vi "Meas Proc QWTB Update Result View Process.vi"(8 "error in":errorcluster, 11 "session in":variant) -> (0 "error out":errorcluster, 3 "QWTB result session out":variant)   [LabVIEW 2018]
doc: "QWTB result viewer: This VI is async. process that will look into current measurement folder. It scans for results header file, then it reads list of the available results for current QWTB algorithm. It fills the result selector by the list of available results.\nThen it tries to load the result data to the table. It also loads descriptions of the table rows which are stored into the QWTB result session. Alternatively it can generate graph of the selected quantity. The decision table vs graph update is made automatically based on the 'QWTB view setup'."
uses:
  Meas Proc QWTB Plot Legend.ctl
  Meas Proc QWTB Viewer Asyn Session.ctl
  Meas Session.ctl
  adc/ADC Session.ctl
  drivers/niScope/niScope Session.ctl
  drivers/niScope/niScope Virtual Channel Config.ctl
  drivers/niScope/niScope Virtual Channel Mode.ctl
  drivers/niScope/niScope Virtual Channel Input Z.ctl
  drivers/niScope/niScope Virtual Channel Coupling.ctl
  drivers/niScope/niScope Type.ctl
  drivers/niScope/niScope Digitizing Process Options.ctl
  drivers/niScope/niScope Data Packet.ctl
  drivers/niScope/niScope Trigger Setup.ctl
  <instrlib>/niScope/Controls/niScope trigger coupling.ctl
  <instrlib>/niScope/Controls/niScope trigger slope.ctl
  drivers/DMM/3458A Digitizer Session.ctl
  drivers/DMM/3458A Virtual Channel Config.ctl
  drivers/Counter/Counter Session.ctl
  drivers/Counter/Counter Type.ctl
  drivers/AWG/AWG Session.ctl
  drivers/AWG/AWG Type.ctl
  drivers/DMM/3458A Sync Mode.ctl
  drivers/DMM/3458A Idn Mode.ctl
  drivers/DMM/3458A Digitizing Low Levels/Configure/Sampling Mode.ctl
  drivers/DMM/3458A Digitizing Process Options.ctl
  drivers/DMM/3458A Data Packet.ctl
  drivers/DMM/3458A Aux Record Data.ctl
  drivers/DMM/3458A Digitizing Low Levels/Configure/Level Setup.ctl
  drivers/DMM/3458A Digitizing Low Levels/Configure/First Sample Trigger.ctl
  drivers/DMM/3458A Aperture Selection Mode.ctl
  drivers/dsdll/DSDLL Session.ctl
  drivers/dsdll/dsdll source distribution/dsdll_instance.ctl
  drivers/dsdll/dsdll source distribution/dsdll_device_record.ctl
  drivers/dsdll/DSDLL Process Config.ctl
  drivers/dsdll/DSDLL Data Packet.ctl
  adc/ADC Type.ctl
  drivers/simulated_adc/SimAdc Config.ctl
  drivers/simulated_adc/SimAdc Channel Cfg.ctl
  adc/ADC On Close Action.ctl
  drivers/Quatsch_driver/QuADCDriver/QuADC Session.ctl
  drivers/Quatsch_driver/QuADCDriver/QuADC Virtual Channel Config.ctl
  drivers/Quatsch_driver/QuADCDriver/QuADC Virtual Channel Mode.ctl
  drivers/Quatsch_driver/QuADCDriver/QuADC Virtual Channel Input Z.ctl
  drivers/Quatsch_driver/QuADCDriver/QuADC Virtual Channel Coupling.ctl
  drivers/Quatsch_driver/QuADCDriver/QuADC Type.ctl
  drivers/Quatsch_driver/QuADCDriver/QuADC Digitizing Process Options.ctl
  drivers/Quatsch_driver/QuADCDriver/QuADC Data Packet.ctl
  drivers/Quatsch_driver/QuADCDriver/QuADC Trigger Setup.ctl
  Meas Sequence Item.ctl
  Meas Sampling Configuration.ctl
  adc/ADC Trig Config.ctl
  adc/ADC Trig Mode Source.ctl
  adc/ADC Trig Coupling.ctl
  adc/ADC Trig Slope.ctl
  Meas Proc QWTB Algorithm Parameter Data.ctl
  Meas Sequence Configuration.ctl
  Meas Range Mode.ctl
  Meas Sampling Rate Mode.ctl
  octave/golpi/mpc/golpi_session_ref.ctl
  Meas Process Config.ctl
  Meas Process Mode.ctl
  Meas Process Raw Config.ctl
  Meas Process Raw Result Mode.ctl
  Meas Proc QWTB Setup.ctl
  Meas Proc QWTB Uncertainty Mode.ctl
  Meas Proc QWTB Multicore Setup.ctl
  Meas Proc QWTB Multicore Type.ctl
  Corrections/Corr Setup.ctl
  Corrections/Corr Tranducer Item.ctl
  Corrections/Corr Digitizers.ctl
  Assist/Assist Panel Setup.ctl
  Meas Proc QWTB Viewer References.ctl
  Meas Proc QWTB Update Flags.ctl
  Meas Proc QWTB Plot Config.ctl
  Meas Proc QWTB Plot Scale Mode.ctl
  varilib/SGUI Assign Multiple Strings With Tags By Label.vi
  octave/golpi/GOLPI Library.lvlibp/Private/Get Variable - polymorph parts/Get String.vi
  octave/golpi/GOLPI Library.lvlibp/Private/Get Variable - polymorph parts/Get Double.vi
  octave/golpi/GOLPI Library.lvlibp/Private/Get Variable - polymorph parts/Get 1D Array Double.vi
  octave/golpi/mpc/GOLPI Multi Process.lvlib
  octave/golpi/GOLPI Library.lvlibp
  varilib/varilib.lvlib
  drivers/niScope/niScope Virtual Digitizer.lvlib
  drivers/DMM/3458A Virtual Digitizer.lvlib
  drivers/Counter/Counter.lvlib
  drivers/AWG/AWG.lvlib
  drivers/DMM/3458A Digitizing Low Levels/3458A Digitizing Low Levels.lvlib
  drivers/dsdll/DSDLL Virtual Digitizer.lvlib
  drivers/Quatsch_driver/QuADCDriver/QuADC Virtual Digitizer.lvlib
  drivers/dsdll/dsdll source distribution/dsdll.lvlib
panel:
  out "user session (memory)":path
  in  "Show legend":T1
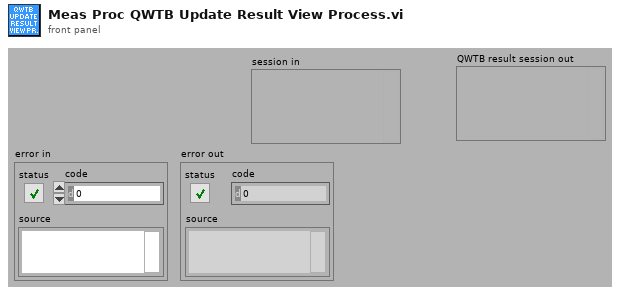
[diagram p1: front panel]
types:
  T1 = typedef "Meas Proc QWTB Plot Legend.ctl" = enum16{"None", "Best", "North", "South", "East", "West", "NorthEast", "NorthWest", "SouthEast", "SouthWest"}
  T2 = typedef "Meas Proc QWTB Viewer Asyn Session.ctl" = cluster{"session":T3, "QWTB result refs":T69, "view setup":T70}
  T3 = typedef "Meas Session.ctl" = cluster{"adc":T4, "sequence":T46[], "sequence setup":T53, "golpi":T56, "processing setup":T57, "corrections":T65, "assist cfg":T68}
  T4 = typedef "ADC Session.ctl" = cluster{"niScope":T5, "3458A":T15, "dsdll":T30, "type":T34, "channel idn str":string[], "aux instr idn str":string[], "modified?":bool, "simadc":T35, "force rst?":bool, "exit mode":T37, "exit dly":dbl, "exit tmr":timestamp, "busy?":bool, "accessed?":bool, "QuADC session":T38}
  T5 = typedef "niScope Virtual Digitizer.lvlib/niScope Session.ctl" = cluster{"channel cfg":T6[], "sessions":refnum<k20>[], "multi cards":bool, "channels":i32, "type":T10, "memory [B/chn]":i32, "ext. clock [Hz]":dbl, "samples count":i64, "use streaming":bool, "proc setup":T11, "sample width [B]":i32, "ranges [V]":dbl[], "trigger setup":T12, "fs [Hz]":dbl, "bitres [bit]":i32}
  T6 = typedef "niScope Virtual Digitizer.lvlib/niScope Virtual Channel Config.ctl" = cluster{"Address":refnum<k15>, "Channel":i32, "Mode":T7, "Input Z":T8, "Coupling":T9, "Range [Vpk]":dbl, "btn clr":bool, "btn up":bool, "btn down":bool}
  T7 = typedef "niScope Virtual Digitizer.lvlib/niScope Virtual Channel Mode.ctl" = enum16{"Single ended", "Unbal. differential", "Differential"}
  T8 = typedef "niScope Virtual Digitizer.lvlib/niScope Virtual Channel Input Z.ctl" = enum16{"1 MOhm", "50 Ohm"}
  T9 = typedef "niScope Virtual Digitizer.lvlib/niScope Virtual Channel Coupling.ctl" = enum16{"AC", "DC", "GND"}
  T10 = typedef "niScope Virtual Digitizer.lvlib/niScope Type.ctl" = enum16{"n/a", "5922"}
  T11 = typedef "niScope Virtual Digitizer.lvlib/niScope Digitizing Process Options.ctl" = cluster{"packet size [smpl]":i64, "current timeout [s]":dbl, "blk2blk timeout [s]":dbl, "event time":timestamp, "temp sampl T [s]":dbl, "data queue":refnum<queue>, "stop notifier":refnum<notifier>, "proc ref":refnum<vi>}
  T12 = typedef "niScope Virtual Digitizer.lvlib/niScope Trigger Setup.ctl" = cluster{"coupling":T13, "level [V]":dbl, "slope":T14, "mode":enum16{"Immediate", "External", "Level"}}
  T13 = typedef "niScope trigger coupling.ctl" = u16
  T14 = typedef "niScope trigger slope.ctl" = i32
  T15 = typedef "3458A Virtual Digitizer.lvlib/3458A Digitizer Session.ctl" = cluster{"channels":T16[], "sync unit":T17, "awg unit":T19, "sync mode":T21, "streaming mode":bool, "idn mode":T22, "sampling mode":T23, "Ts [s]":dbl, "sample memory [B]":i32, "proc setup":T24, "sample size [B]":i32, "sample count":i32, "aux data":T26, "ranges [V]":dbl[], "aperture [s]":dbl, "LEVEL trigger":T27, "trigger mode":T28, "measure temp.?":bool, "disp mesages":string[], "shared bus?":bool, "disable display?":bool, "aper mode":T29, "aper rules":dbl[][]}
  T16 = typedef "3458A Virtual Digitizer.lvlib/3458A Virtual Channel Config.ctl" = cluster{"VISA":refnum<visa-resource-name>, "Range [Vpk]":dbl, "btn clr":bool, "btn up":bool, "btn down":bool}
  T17 = typedef "Counter.lvlib/Counter Session.ctl" = cluster{"VISA":refnum<visa-resource-name>, "type":T18}
  T18 = typedef "Counter.lvlib/Counter Type.ctl" = enum16{"Picotest U6200A", "dummy"}
  T19 = typedef "AWG.lvlib/AWG Session.ctl" = cluster{"type":T20, "VISA":refnum<visa-resource-name>, "enable 10MHz ref":bool}
  T20 = typedef "AWG.lvlib/AWG Type.ctl" = enum16{"Agilent 331xxA to 332xxA", "Agilent 335xxA to 336xxA", "Tektronix AFG3101C", "dummy"}
  T21 = typedef "3458A Virtual Digitizer.lvlib/3458A Sync Mode.ctl" = enum16{"MASTER-SLAVE, MASTER clocked by TIMER", "MASTER-SLAVE, MASTER clocked by AWG", "ALL clocked by AWG", "MASTER-SLAVE, ALL clocked by TIMER", "ALL clocked by AWG with DFLL"}
  T22 = typedef "3458A Virtual Digitizer.lvlib/3458A Idn Mode.ctl" = enum16{"Auto", "Sequential (chn A, chn B, ...)", "From calibration string"}
  T23 = typedef "3458A Virtual Digitizer.lvlib/3458A Digitizing Low Levels.lvlib/Sampling Mode.ctl" = enum16{"DCV", "DSDC", "DSAC"}
  T24 = typedef "3458A Virtual Digitizer.lvlib/3458A Digitizing Process Options.ctl" = cluster{"channel id":i32, "packet size [smpl]":i32, "current timeout [s]":dbl, "blk2blk timeout [s]":dbl, "event time":timestamp, "stop notifier":refnum<notifier>, "data queues":refnum<queue>[], "proc refs":refnum<vi>[], "bus semaphore":T25}
  T25 = typedef "Semaphore RefNum" = refnum<k1>
  T26 = typedef "3458A Virtual Digitizer.lvlib/3458A Aux Record Data.ctl" = cluster{"channel id":i32, "valid?":bool[], "gain [V]":dbl[], "timestamp [s]":dbl[], "Ts [s]":dbl, "abs timestamp":timestamp, "t [deg C]":dbl[]}
  T27 = typedef "3458A Virtual Digitizer.lvlib/3458A Digitizing Low Levels.lvlib/Level Setup.ctl" = cluster{"edge":enum16{"POS", "NEG"}, "level [V]":dbl, "coupling":enum16{"DC", "AC"}}
  T28 = typedef "3458A Virtual Digitizer.lvlib/3458A Digitizing Low Levels.lvlib/First Sample Trigger.ctl" = enum16{"AUTO", "EXT", "SYN", "SGL", "HOLD", "LEVEL"}
  T29 = typedef "3458A Virtual Digitizer.lvlib/3458A Aperture Selection Mode.ctl" = enum16{"Manual", "Maximum", "Table"}
  T30 = typedef "DSDLL Virtual Digitizer.lvlib/DSDLL Session.ctl" = cluster{"dsdll":T31, "channels":i32, "device id":i32, "channel idns":string[], "proc setup":T33, "samples count":i32, "fs [Hz]":dbl}
  T31 = typedef "dsdll.lvlib/dsdll_instance.ctl" = cluster{"dsdll path":path, "dsdll handle":u8[], "output devices":T32[], "capture devices":T32[]}
  T32 = typedef "dsdll.lvlib/dsdll_device_record.ctl" = cluster{"guid":u8[], "name":string}
  T33 = typedef "DSDLL Virtual Digitizer.lvlib/DSDLL Process Config.ctl" = cluster{"packet size [smpl]":i32, "current timeout [s]":dbl, "blk2blk timeout [s]":dbl, "event time":timestamp, "data queue":refnum<queue>, "stop notifier":refnum<notifier>, "proc ref":refnum<vi>}
  T34 = typedef "ADC Type.ctl" = enum16{"niScope", "3458A", "DirectSound DLL", "dummy", "QuADC"}
  T35 = typedef "SimAdc Config.ctl" = cluster{"channels":T36[], "range [V]":dbl, "Ts step [s]":dbl, "time [s]":dbl, "fs [Hz]":dbl, "count":i64, "smpl offset":i64, "set count":i64, "bit res":i32}
  T36 = typedef "SimAdc Channel Cfg.ctl" = cluster{"harmonics":dbl[][], "btn clear":bool, "noise":dbl, "fundamental [Hz]":dbl}
  T37 = typedef "ADC On Close Action.ctl" = enum16{"Immediate reset", "Delayed reset"}
  T38 = typedef "QuADC Virtual Digitizer.lvlib/QuADC Session.ctl" = cluster{"channel cfg":T39[], "sessions":refnum<k5>[], "multi cards":bool, "channels":i32, "type":T43, "memory [B/chn]":i32, "ext. clock [Hz]":dbl, "samples count":i64, "use streaming":bool, "proc setup":T44, "sample width [B]":i32, "ranges [V]":dbl[], "trigger setup":T45, "fs [Hz]":dbl, "bitres [bit]":i32}
  T39 = typedef "QuADC Virtual Digitizer.lvlib/QuADC Virtual Channel Config.ctl" = cluster{"Channel":i32, "Mode":T40, "Input Z":T41, "Coupling":T42, "Range [Vpk]":dbl, "btn clr":bool, "btn up":bool, "btn down":bool, "IP address A":u8, "IP address B":u8, "IP address C":u8, "IP address D":u8, "Port":u16, "Number of JJ":u32, "Clock fr. (Hz)":dbl}
  T40 = typedef "QuADC Virtual Digitizer.lvlib/QuADC Virtual Channel Mode.ctl" = enum16{"Single ended", "Unbal. differential", "Differential"}
  T41 = typedef "QuADC Virtual Digitizer.lvlib/QuADC Virtual Channel Input Z.ctl" = enum16{"1 MOhm", "50 Ohm"}
  T42 = typedef "QuADC Virtual Digitizer.lvlib/QuADC Virtual Channel Coupling.ctl" = enum16{"AC", "DC", "GND"}
  T43 = typedef "QuADC Virtual Digitizer.lvlib/QuADC Type.ctl" = enum16{"n/a", "v1"}
  T44 = typedef "QuADC Virtual Digitizer.lvlib/QuADC Digitizing Process Options.ctl" = cluster{"packet size [smpl]":i64, "current timeout [s]":dbl, "blk2blk timeout [s]":dbl, "event time":timestamp, "temp sampl T [s]":dbl, "data queue":refnum<queue>, "stop notifier":refnum<notifier>, "proc ref":refnum<vi>}
  T45 = typedef "QuADC Virtual Digitizer.lvlib/QuADC Trigger Setup.ctl" = cluster{"coupling":T13, "level [V]":dbl, "slope":T14, "mode":enum16{"Immediate", "External", "Level"}}
  T46 = typedef "Meas Sequence Item.ctl" = cluster{"config":T47, "data file path":path, "header file path":path, "group id":i32, "average id":i32, "group done?":bool, "adc modified?":bool, "source modified?":bool, "progress [%]":dbl, "groups cnt":i32, "average cnt":i32, "data file relative path":string, "meas root path":path, "calculate?":bool}
  T47 = typedef "Meas Sampling Configuration.ctl" = cluster{"fs [Hz]":dbl, "count [smpl]":i64, "aperture [s]":dbl, "trigger":T48, "ranges [Vpk]":dbl[], "QWTB parameters":T52[]}
  T48 = typedef "ADC Trig Config.ctl" = cluster{"source":T49, "level [V]":dbl, "coupling":T50, "slope":T51}
  T49 = typedef "ADC Trig Mode Source.ctl" = enum16{"Immediate", "External", "Level"}
  T50 = typedef "ADC Trig Coupling.ctl" = enum16{"DC", "AC"}
  T51 = typedef "ADC Trig Slope.ctl" = enum16{"POS", "NEG"}
  T52 = typedef "Meas Proc QWTB Algorithm Parameter Data.ctl" = cluster{"name":string, "numerics":dbl[], "strings":string[]}
  T53 = typedef "Meas Sequence Configuration.ctl" = cluster{"group setups":T47[], "average cycles":i32, "range mode":T54, "fs mode":T55, "rng even":dbl, "rng odd":dbl, "folder":path, "name base":string, "meas id":i32, "settle [s]":dbl}
  T54 = typedef "Meas Range Mode.ctl" = enum16{"Keep defaults", "Set All channels", "Set Odd and Even channels"}
  T55 = typedef "Meas Sampling Rate Mode.ctl" = enum16{"Frequency", "Period"}
  T56 = typedef "GOLPI Multi Process.lvlib/golpi_session_ref.ctl" = refnum<vi>
  T57 = typedef "Meas Process Config.ctl" = cluster{"mode":T58, "call after avgs?":bool, "calculate?":bool, "raw mode":T59, "QWTB":T61}
  T58 = typedef "Meas Process Mode.ctl" = enum16{"Raw", "QWTB"}
  T59 = typedef "Meas Process Raw Config.ctl" = cluster{"command":string, "result mode":T60, "res variable":string}
  T60 = typedef "Meas Process Raw Result Mode.ctl" = enum16{"Display console output (only Octave)", "Display string variable", "Display result file %respath%"}
  T61 = typedef "Meas Proc QWTB Setup.ctl" = cluster{"QWTB path":path, "alg filter path":string, "alg ids":string[], "alg parameters":string[], "parsed parameters":T52[], "selected alg id":string, "selected unc mode":T62, "qwtb mcc":i32, "qwtb timeout":i32, "qwtb covg":dbl, "qwtb ofs":i64, "qwtb lim data":i64, "multicore":T63, "unc once?":bool}
  T62 = typedef "Meas Proc QWTB Uncertainty Mode.ctl" = enum16{"None", "GUF", "Monte Carlo"}
  T63 = typedef "Meas Proc QWTB Multicore Setup.ctl" = cluster{"jobs folder":path, "cores":i32, "max jobs":i32, "mode":T64}
  T64 = typedef "Meas Proc QWTB Multicore Type.ctl" = enum16{"Singlecore", "Multicore", "Multistation"}
  T65 = typedef "Corr Setup.ctl" = cluster{"transducers":cluster{"channels":T66[], "last path":path}, "digitizer":T67}
  T66 = typedef "Corr Tranducer Item.ctl" = cluster{"Path":path, "Ratio:":string, "Name:":string, "btn rem":bool, "btn up":bool, "btn down":bool, "s.n.:":string, "btn open":bool, "ratio o/i":dbl, "chn hi":u16, "chn lo":u16, "Phase index":i32}
  T67 = typedef "Corr Digitizers.ctl" = cluster{"last path":path, "channel paths":path[], "channel idns":string[], "correction name":string, "channel names":string[], "folders to copy":path[], "channel valid":bool[], "correction path":path, "correction rel path":string, "rel folders to copy":string[]}
  T68 = typedef "Assist Panel Setup.ctl" = cluster{"P":i32, "Q":i32, "rel shift":dbl, "ref freq":dbl, "min fs":dbl, "max fs tol":dbl, "min int":dbl, "max int":dbl, "max err":dbl, "max timeout":dbl}
  T69 = typedef "Meas Proc QWTB Viewer References.ctl" = cluster{"tc result":refnum<vi>, "qwtb results tbl":refnum<vi>, "qwtb maxdim":refnum<vi>, "qwtb unc":refnum<vi>, "qwtb order":refnum<vi>, "qwtb maxarr":refnum<vi>, "qwtb res sel":refnum<vi>, "qwtb res info":refnum<vi>, "descriptions":string[], "var names":string[], "channel indexes":i32[], "qwtb ref chn":refnum<vi>, "qwtb ph unit":refnum<vi>, "qwtb alg sel":refnum<vi>, "qwtb meas sel":refnum<vi>, "qwtb ssn info":refnum<vi>, "last session":path, "qwtb qu list":refnum<vi>}
  T70 = typedef "Meas Proc QWTB Update Flags.ctl" = cluster{"new result":bool, "show graph":bool, "plot setup":T71, "new session":bool}
  T71 = typedef "Meas Proc QWTB Plot Config.ctl" = cluster{"X-axis style":T72, "Y-axis style":T72, "Show legend":T1, "Grid on":bool, "Box on":bool, "show all chn":bool}
  T72 = typedef "Meas Proc QWTB Plot Scale Mode.ctl" = enum16{"Linear", "Log"}
  T73 = typedef "GOLPI Library.lvlibp/GOLPI reference Type Def.ctl" = cluster{"pipe handle":T74, "fast read timeout [ms]":u32, "fast read settle time [ms]":u32, "fast read to multiple [ms]":u32, "max elements per input line":u32, "slow read timeout [ms]":u32, "stdin double format specifier":string, "max elements per stdout output column":u32, "console mode bitstream":bool, "bitstream first read timeout [ms]":u32, "bitstream read timeout [ms]":u32, "struct transfer possible":bool, "matlab mode":bool}
  T74 = typedef "GOLPI Library.lvlibp/LV Process library.lvlib/Pipe Handle.ctl" = cluster{"lv_proc.dll file path":path, "process instance handle":u32[], "debug mode":bool, "debug data":cluster{"time":timestamp, "stdin":bool, "data":string}[]}
  T75 = typedef "Meas Proc QWTB View Max Dim.ctl" = enum16{"Scalar", "Vector", "Matrix"}
  T76 = typedef "Meas Proc QWTB View Group Mode.ctl" = enum16{"Group quantities", "Group phases"}
  T77 = typedef "Meas Proc QWTB View Uncertainty Mode.ctl" = enum16{"None", "val ± unc", "[val; unc]"}
  T78 = typedef "Meas Proc QWTB View Phase Mode.ctl" = enum16{"± pi [rad]", "0 - 2*pi [rad]", "±180 [deg]", "0 - 360 [deg]"}
  T79 = typedef "LVRowAndColumnTypeDef.ctl" = cluster{"Row":i32, "Column":i32}
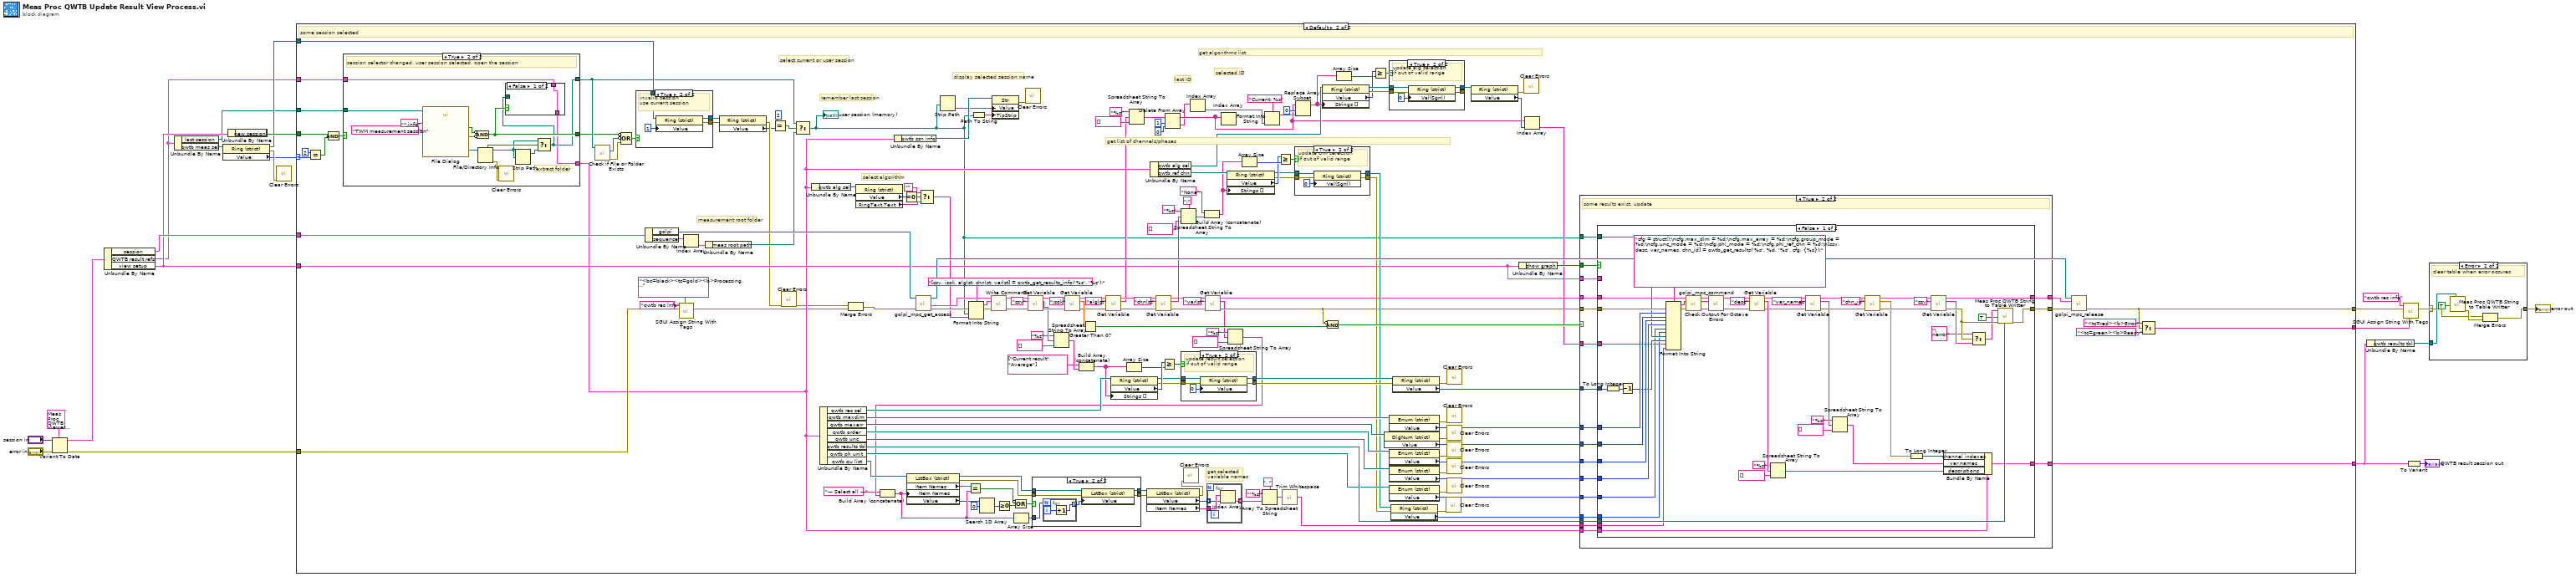
[diagram p0: block diagram]
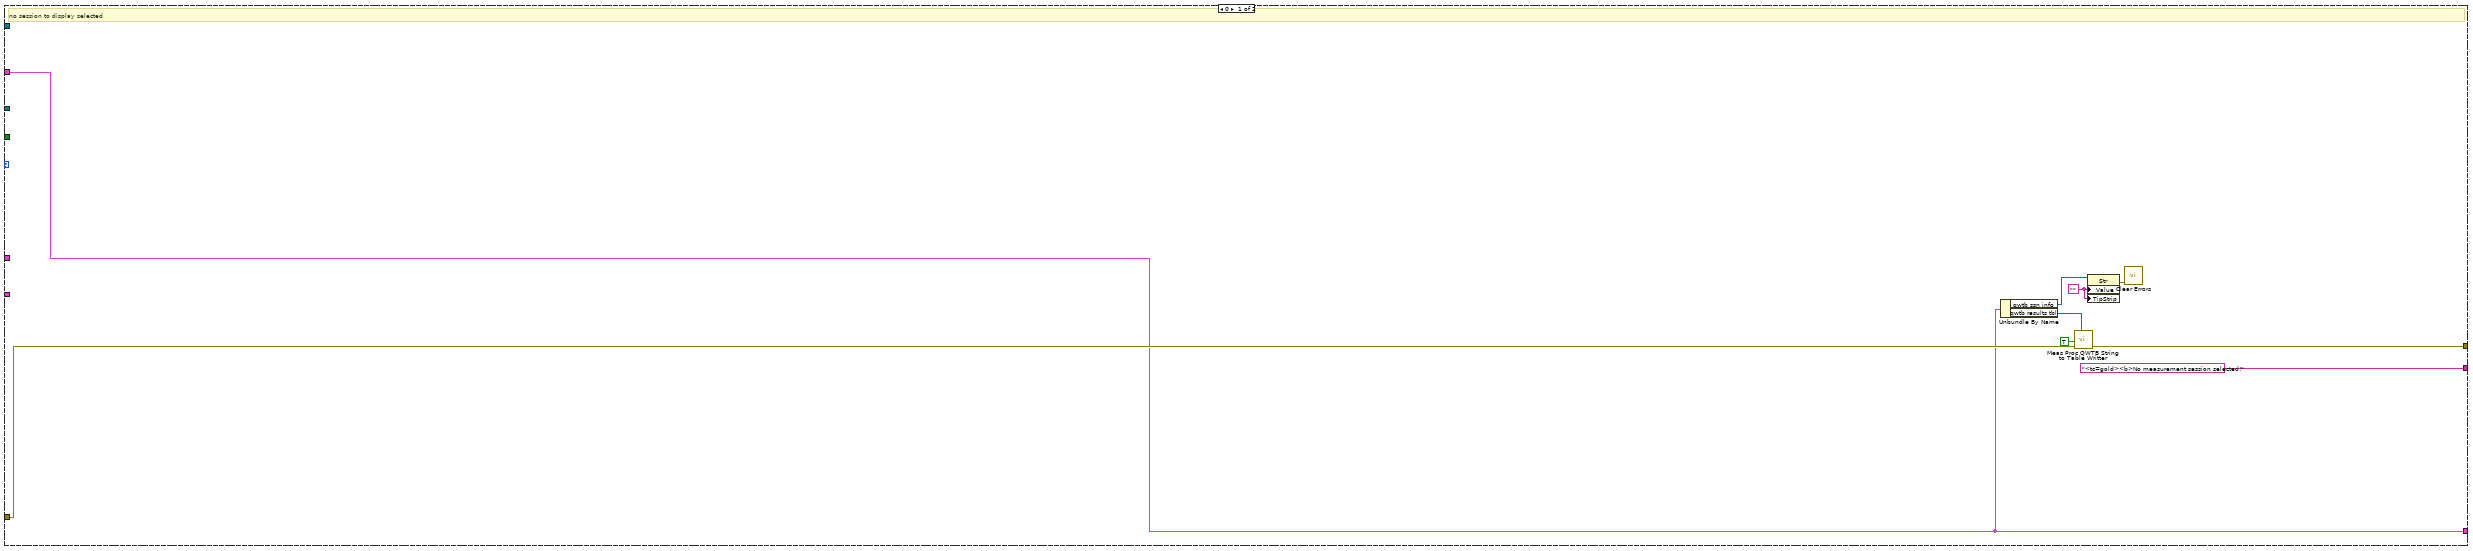
[diagram p3: hidden frame]
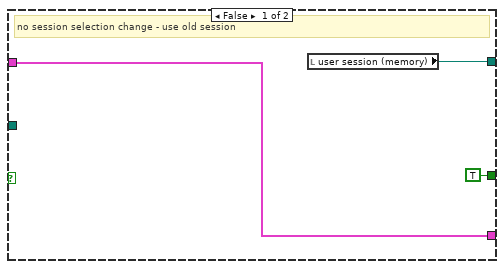
[diagram p6: hidden frame]
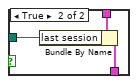
[diagram p7: hidden frame]
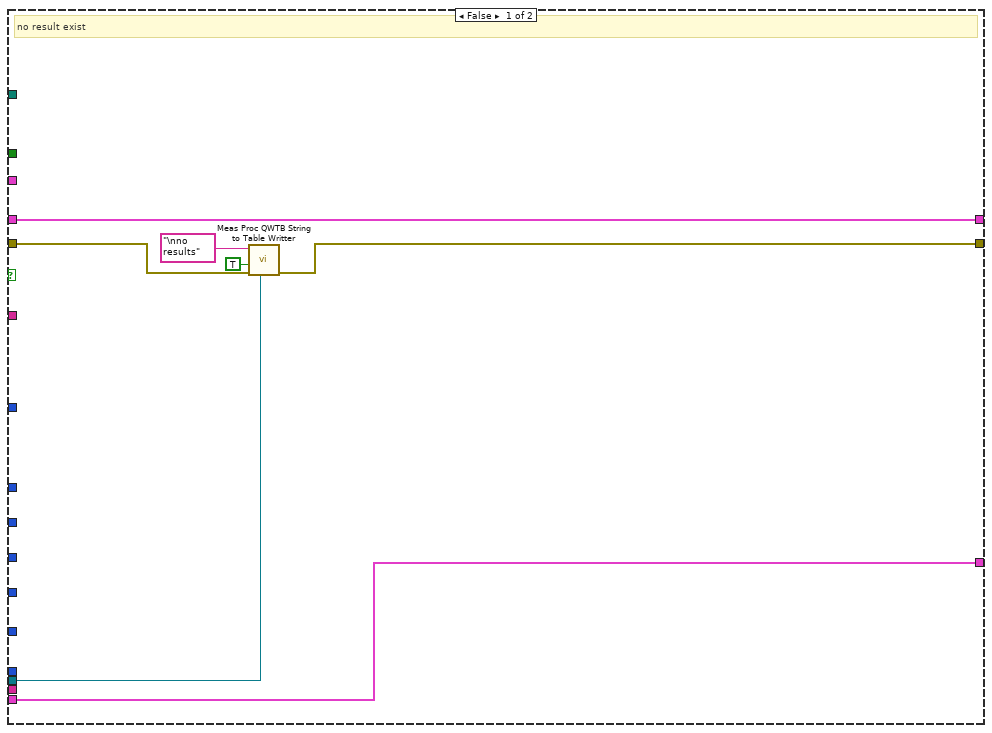
[diagram p10: hidden frame]
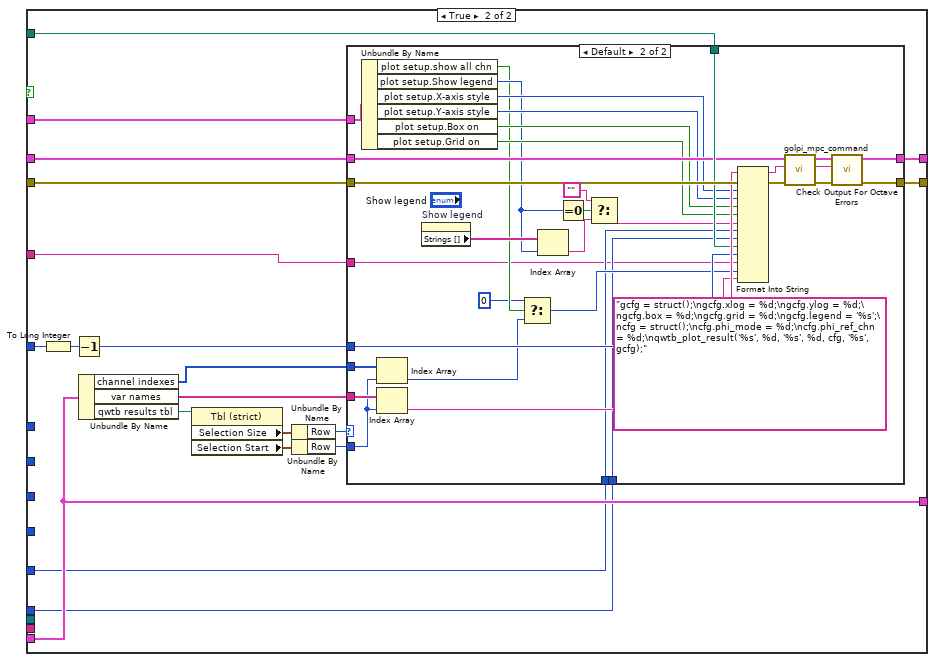
[diagram p11: hidden frame]
diagram:
  n1 = Variant To Data(error in="error in", type=T2 {"session"={"adc"={"niScope"={"channel cfg"=[], "sessions"=[], "multi cards"=FALSE, "channels"=0, "type"=enum."n/a", "memory [B/chn]"=0, "ext. clock [Hz]"=0.0, "samples count"=0, "use streaming"=FALSE, "proc setup"={"packet size [smpl]"=0, "current timeout [s]"=0.0, "blk2blk timeout [s]"=0.0, "event time"=timestamp(0 s since 1904-01-01), "temp sampl T [s]"=0.0, "data queue"=refnum, "stop notifier"=refnum, "proc ref"=refnum}, "sample width [B]"=0, "ranges [V]"=[], "trigger setup"={"coupling"=1, "level [V]"=0.0, "slope"=0, "mode"=enum."Immediate"}, "fs [Hz]"=0.0, "bitres [bit]"=0}, "3458A"={"channels"=[], "sync unit"={"VISA"="", "type"=enum."Picotest U6200A"}, "awg unit"={"type"=enum."Agilent 331xxA to 332xxA", "VISA"="", "enable 10MHz ref"=FALSE}, "sync mode"=enum."MASTER-SLAVE, MASTER clocked by TIMER", "streaming mode"=FALSE, "idn mode"=enum."Auto", "sampling mode"=enum."DCV", "Ts [s]"=0.0, "sample memory [B]"=0, "proc setup"={"channel id"=0, "packet size [smpl]"=0, "current timeout [s]"=0.0, "blk2blk timeout [s]"=0.0, "event time"=timestamp(0 s since 1904-01-01), "stop notifier"=refnum, "data queues"=[], "proc refs"=[], "bus semaphore"=refnum}, "sample size [B]"=0, "sample count"=0, "aux data"={"channel id"=0, "valid?"=[], "gain [V]"=[], "timestamp [s]"=[], "Ts [s]"=0.0, "abs timestamp"=timestamp(0 s since 1904-01-01), "t [deg C]"=[]}, "ranges [V]"=[], "aperture [s]"=0.0, "LEVEL trigger"={"edge"=enum."POS", "level [V]"=0.0, "coupling"=enum."DC"}, "trigger mode"=enum."AUTO", "measure temp.?"=FALSE, "disp mesages"=[], "shared bus?"=FALSE, "disable display?"=FALSE, "aper mode"=enum."Manual", "aper rules"=[]}, "dsdll"={"dsdll"={"dsdll path"=path "", "dsdll handle"=[], "output devices"=[], "capture devices"=[]}, "channels"=0, "device id"=0, "channel idns"=[], "proc setup"={"packet size [smpl]"=0, "current timeout [s]"=0.0, "blk2blk timeout [s]"=0.0, "event time"=timestamp(0 s since 1904-01-01), "data queue"=refnum, "stop notifier"=refnum, "proc ref"=refnum}, "samples count"=0, "fs [Hz]"=0.0}, "type"=enum."niScope", "channel idn str"=[], "aux instr idn str"=[], "modified?"=FALSE, "simadc"={"channels"=[], "range [V]"=0.0, "Ts step [s]"=0.0, "time [s]"=0.0, "fs [Hz]"=0.0, "count"=0, "smpl offset"=0, "set count"=0, "bit res"=0}, "force rst?"=FALSE, "exit mode"=enum."Immediate reset", "exit dly"=0.0, "exit tmr"=timestamp(0 s since 1904-01-01), "busy?"=FALSE, "accessed?"=FALSE, "QuADC session"={"channel cfg"=[], "sessions"=[], "multi cards"=FALSE, "channels"=0, "type"=enum."n/a", "memory [B/chn]"=0, "ext. clock [Hz]"=0.0, "samples count"=0, "use streaming"=FALSE, "proc setup"={"packet size [smpl]"=0, "current timeout [s]"=0.0, "blk2blk timeout [s]"=0.0, "event time"=timestamp(0 s since 1904-01-01), "temp sampl T [s]"=0.0, "data queue"=refnum, "stop notifier"=refnum, "proc ref"=refnum}, "sample width [B]"=0, "ranges [V]"=[], "trigger setup"={"coupling"=0, "level [V]"=0.0, "slope"=0, "mode"=enum."Immediate"}, "fs [Hz]"=0.0, "bitres [bit]"=0}}, "sequence"=[], "sequence setup"={"group setups"=[], "average cycles"=0, "range mode"=enum."Keep defaults", "fs mode"=enum."Frequency", "rng even"=0.0, "rng odd"=0.0, "folder"=path "", "name base"="", "meas id"=0, "settle [s]"=0.0}, "golpi"=refnum, "processing setup"={"mode"=enum."Raw", "call after avgs?"=FALSE, "calculate?"=FALSE, "raw mode"={"command"="", "result mode"=enum."Display console output (only Octave)", "res variable"=""}, "QWTB"={"QWTB path"=path "", "alg filter path"="", "alg ids"=[], "alg parameters"=[], "parsed parameters"=[], "selected alg id"="", "selected unc mode"=enum."None", "qwtb mcc"=0, "qwtb timeout"=0, "qwtb covg"=0.0, "qwtb ofs"=0, "qwtb lim data"=0, "multicore"={"jobs folder"=path "", "cores"=0, "max jobs"=0, "mode"=enum."Singlecore"}, "unc once?"=FALSE}}, "corrections"={"transducers"={"channels"=[], "last path"=path ""}, "digitizer"={"last path"=path "", "channel paths"=[], "channel idns"=[], "correction name"="", "channel names"=[], "folders to copy"=[], "channel valid"=[], "correction path"=path "", "correction rel path"="", "rel folders to copy"=[]}}, "assist cfg"={"P"=0, "Q"=0, "rel shift"=0.0, "ref freq"=0.0, "min fs"=0.0, "max fs tol"=0.0, "min int"=0.0, "max int"=0.0, "max err"=0.0, "max timeout"=0.0}}, "QWTB result refs"={"tc result"=refnum, "qwtb results tbl"=refnum, "qwtb maxdim"=refnum, "qwtb unc"=refnum, "qwtb order"=refnum, "qwtb maxarr"=refnum, "qwtb res sel"=refnum, "qwtb res info"=refnum, "descriptions"=[], "var names"=[], "channel indexes"=[], "qwtb ref chn"=refnum, "qwtb ph unit"=refnum, "qwtb alg sel"=refnum, "qwtb meas sel"=refnum, "qwtb ssn info"=refnum, "last session"=path "", "qwtb qu list"=refnum}, "view setup"={"new result"=FALSE, "show graph"=FALSE, "plot setup"={"X-axis style"=enum."Linear", "Y-axis style"=enum."Linear", "Show legend"=enum."None", "Grid on"=FALSE, "Box on"=FALSE, "show all chn"=FALSE}, "new session"=FALSE}} ("Cluster"), Variant="session in") -> (data=w18:T2, error out=w16:errorcluster)
  n2 = Unbundle By Name(w18) -> ("session"=w17:T3, "QWTB result refs"=w9:T69, "view setup"=w15:T70)
  n3 = Unbundle By Name(w9) -> ("last session"=w10:path, "qwtb meas sel"=w14:refnum<vi>)
  n4 = property class="Ring (strict)"(reference=w14) -> (reference out=w12:refnum<vi>, error out=w11:errorcluster, "Value"=w8:u16)  [unwired: 1 in]
  n5 = Unbundle By Name(w15) -> ("new session"=w13:bool)
  n6 = call <vilib>:"Clear Errors.vi"("error in (no error)"=w11) -> ()  [unwired: 5 in, 2 out]
  n7 = case shown="Default" w8 {
    selector: w8 -> [_ w73]
    tunnel: [w29 w72] -> w6
    tunnel: [w28 w64] -> w2
    tunnel: w17 -> [_ w150]
    tunnel: w16 -> [w30 w149]
    tunnel: w15 -> [_ w102]
    tunnel: w13 -> [_ w101]
    tunnel: w12 -> [_ w97]
    tunnel: w10 -> [_ w86]
    tunnel: w9 -> [w28 w85]
    tunnel: ["<tc=gold><b>No measurement session selected!" ("string (empty)") w71] -> w5
    frame 0 {
      w24 = "" ("Value")
      # "no session to display selected"
      n8 = Unbundle By Name(w28) -> ("qwtb ssn info"=w25:refnum<vi>, "qwtb results tbl"=w27:refnum<vi>)
      n9 = call "Meas Proc QWTB String to Table Writter.vi"("param table ref"=w27, "error in"=w30, "force data update? (False)"=TRUE) -> ("error out"=w29:errorcluster)  [unwired: 7 in, 1 out]
      n10 = property class="Str"(reference=w25, "Value"=w24, "TipStrip"=w24) -> (error out=w23:errorcluster)  [unwired: 1 in, 1 out]
      n11 = call <vilib>:"Clear Errors.vi"("error in (no error)"=w23) -> ()  [unwired: 5 in, 2 out]
    }
    frame Default {
      # "get selected\nvariable names"
      # "last ID"
      # "selected ID"
      # "display selected session name"
      # "remember last session"
      # "select current or user session"
      # "select algorithm"
      # "get list of channels/phases"
      # "get algorithms list"
      # "measurement root folder"
      # "some session selected"
      n12 = Equal?(x=u16 2, y=w73) -> (x = y?=w77:bool)
      n13 = Compound Arithmetic op=AND(w101, w77) -> (w100:bool)
      n14 = case shown="True" w100 {
        tunnel: [w228 w230] -> w96
        tunnel: [TRUE w231] -> w95
        tunnel: w86 -> [_ w232]
        tunnel: w85 -> [w226 w233]
        tunnel: [w226 w229] -> w84
        frame False {
          # "no session selection change - use old session"
          n15 = local read "user session (memory)"() -> (w228:path)
        }
        frame True {
          # "extract folder"
          # "session selector changed, user session selected, open the session"
          n16 = call "File Dialog"("start path"=w232, "pattern (all files)"="*.info", "pattern label"="TWM measurement session") -> ("selected path"=w238:path, "cancelled"=w240:bool, "error out"=w239:errorcluster)  [unwired: 9 in, 1 out]
          n17 = Compound Arithmetic op=AND(invert w240, invert w239) -> (w231:bool)
          n18 = File/Directory Info(path=w238) -> (path out=w236:path, directory=w237:bool, error out=w234:errorcluster)  [unwired: 1 in, 4 out]
          n19 = call <vilib>:"Clear Errors.vi"("error in (no error)"=w234) -> ()  [unwired: 5 in, 2 out]
          n20 = Strip Path(path=w236) -> (stripped path=w235:path)  [unwired: 1 out]
          n21 = Select(t=w236, s=w237, f=w235) -> (s? t:f=w230:path)
          n22 = case shown="False" w231 {
            tunnel: w233 -> [w243 w246]
            tunnel: w230 -> [_ w245]
            tunnel: [w243 w244] -> w229
            frame False {
            }
            frame True {
              n23 = Bundle By Name(cluster=w246, "last session"=w245) -> (w244:T69)
            }
          }
        }
      }
      n24 = call <vilib>:"Check if File or Folder Exists.vi"("path"=w96) -> ("error out"=w93:errorcluster, "file or folder exists?"=w94:bool)  [unwired: 8 in, 1 out]
      n25 = Compound Arithmetic op=OR(invert w95, invert w94, w93) -> (w92:bool)
      n26 = case shown="True" w92 {
        tunnel: w97 -> [w221 w225]
        tunnel: [w221 w223] -> w98
        tunnel: [_ w222] -> w91
        frame False {
        }
        frame True {
          # "invalid session\nuse current session"
          n27 = property class="Ring (strict)"(reference=w225, "Value"=u16 1) -> (reference out=w223:refnum<vi>, error out=w222:errorcluster)  [unwired: 1 in]
        }
      }
      n28 = Unbundle By Name(w150) -> ("golpi"=w205:T56, "sequence"=w207:T46[])
      n29 = call-poly "SGUI Assign String With Tags.vi"("error in"=w149, "label(s) (empty)"="qwtb res info", "string (empty)"="<bc=black><tc=gold><b>Processing...") -> ("error out"=w83:errorcluster)  [unwired: 7 in, 1 out]
      n30 = Index Array(array=w207) -> (element=w206:T46)  [unwired: 1 in]
      n31 = Unbundle By Name(w206) -> ("meas root path"=w99:path)
      n32 = property class="Ring (strict)"(reference=w98, error in=w91) -> (error out=w90:errorcluster, "Value"=w76:u16)  [unwired: 1 out]
      n33 = Equal?(x=u16 2, y=w76) -> (x = y?=w75:bool)
      n34 = call <vilib>:"Clear Errors.vi"("error in (no error)"=w90) -> ("error out"=w81:errorcluster)  [unwired: 5 in, 1 out]
      n35 = Select(t=w96, s=w75, f=w99) -> (s? t:f=w80:path)
      "user session (memory)" <- w80
      n36 = Unbundle By Name(w84) -> ("qwtb alg sel"=w108:refnum<vi>)
      n37 = Unbundle By Name(w84) -> ("qwtb res sel"=w188:refnum<vi>, "qwtb maxdim"=w174:refnum<vi>, "qwtb maxarr"=w173:refnum<vi>, "qwtb order"=w172:refnum<vi>, "qwtb unc"=w171:refnum<vi>, "qwtb results tbl"=w162:refnum<vi>, "qwtb ph unit"=w152:refnum<vi>, "qwtb qu list"=w48:refnum<vi>)
      n38 = Merge Errors(w81, w83) -> (w82:errorcluster)
      n39 = property class="Ring (strict)"(reference=w108) -> ("Value"=w107:u16, "RingText.Text"=w105:string)  [unwired: 1 in, 2 out]
      n40 = Unbundle By Name(w84) -> ("qwtb ssn info"=w89:refnum<vi>)
      n41 = Equal To 0?(x=w107) -> (x = 0?=w106:bool)
      n42 = call "golpi_mpc_get_access.vi"("error in"=w82, "golpi session ref"=w205) -> ("error out"=w203:errorcluster, "GOLPI ref out"=w204:T73, "golpi session ref out (copy)"=w159:T56)  [unwired: 4 in, 3 out]
      n43 = Select(t="", s=w106, f=w105) -> (s? t:f=w103:string)
      n44 = Strip Path(path=w80) -> (name=w88:string)  [unwired: 1 out]
      n45 = Format Into String(format string="[csv, isok, alglst, chnlst, varlst] = qwtb_get_results_info('%s', '%s');", error in=w203, w80, w103) -> (resulting string=w201:string, error out=w202:errorcluster)  [unwired: 1 in]
      n46 = Path To String(path=w80) -> (string=w79:string)
      n47 = call "Write Command.vi"("error in"=w202, "command"=w201, "GOLPI ref. in"=w204) -> ("error out"=w199:errorcluster, "GOLPI ref. out"=w198:T73)  [unwired: 7 in]
      n48 = property class="Str"(reference=w89, "Value"=w88, "TipStrip"=w79) -> (error out=w87:errorcluster)  [unwired: 1 in, 1 out]
      n49 = call <vilib>:"Clear Errors.vi"("error in (no error)"=w87) -> ()  [unwired: 5 in, 2 out]
      n50 = call-poly "Get Variable.vi"("error in"=w199, "variable name"="csv", "GOLPI ref. in"=w198) -> ("error out"=w196:errorcluster, "value"=w192:string, "GOLPI ref. out"=w194:T73)  [unwired: 6 in]
      n51 = Spreadsheet String To Array(format string="%s", spreadsheet string=w192, array type (2D Dbl)=string[] []) -> (array=w190:string[])  [unwired: 1 in]
      n52 = call-poly "Get Variable.vi"("error in"=w196, "variable name"="isok", "GOLPI ref. in"=w194) -> ("error out"=w130:errorcluster, "value"=w180:dbl, "GOLPI ref. out"=w127:T73)  [unwired: 6 in]
      n53 = Build Array (concatenate)(string[] ["Current result", "Average"], w190) -> (w187:string[])
      n54 = Greater Than 0?(x=w180) -> (x > 0?=w179:bool)
      n55 = call-poly "Get Variable.vi"("error in"=w130, "variable name"="alglst", "GOLPI ref. in"=w127) -> ("error out"=w129:errorcluster, "value"=w123:string, "GOLPI ref. out"=w128:T73)  [unwired: 6 in]
      n56 = property class="Ring (strict)"(reference=w188, "Strings []"=w187) -> (reference out=w183:refnum<vi>, error out=w182:errorcluster, "Value"=w186:u16)  [unwired: 1 in]
      n57 = Array Size(array=w187) -> (size(s)=w185:i32)
      n58 = Spreadsheet String To Array(format string="%s", spreadsheet string=w123, array type (2D Dbl)=string[] []) -> (array=w70:string[])  [unwired: 1 in]
      n59 = Unbundle By Name(w84) -> ("qwtb alg sel"=w113:refnum<vi>, "qwtb ref chn"=w141:refnum<vi>)
      n60 = call-poly "Get Variable.vi"("error in"=w129, "variable name"="chnlst", "GOLPI ref. in"=w128) -> ("error out"=w56:errorcluster, "value"=w145:string, "GOLPI ref. out"=w54:T73)  [unwired: 6 in]
      n61 = Greater Or Equal?(x=w186, y=w185) -> (x >= y?=w184:bool)
      n62 = Delete From Array(array=w70, length=1, index=0) -> (deleted portion=w67:string[], array with subset deleted=w69:string[])
      n63 = Spreadsheet String To Array(delimiter (Tab)=";", format string="%s", spreadsheet string=w145, array type (2D Dbl)=string[] []) -> (array=w140:string[])
      n64 = case shown="True" w184 {
        tunnel: w183 -> [w393 w399]
        tunnel: w182 -> [w394 w398]
        tunnel: [w394 w396] -> w178
        tunnel: [w393 w395] -> w177
        frame False {
        }
        frame True {
          # "update result selection\nif out of valid range"
          n65 = property class="Ring (strict)"(reference=w399, error in=w398, "Value"=u16 0) -> (reference out=w395:refnum<vi>, error out=w396:errorcluster)
        }
      }
      n66 = Index Array(array=w67) -> (element=w66:string)  [unwired: 1 in]
      n67 = Build Array (concatenate)("None" ("delimiter (Tab)"), w140) -> (w138:string[])
      n68 = call-poly "Get Variable.vi"("error in"=w56, "variable name"="varlst", "GOLPI ref. in"=w54) -> ("error out"=w55:errorcluster, "value"=w49:string, "GOLPI ref. out"=w53:T73)  [unwired: 6 in]
      n69 = Index Array(array=w69) -> ()  [unwired: 1 in, 1 out]
      n70 = property class="Ring (strict)"(reference=w141, "Strings []"=w138) -> (reference out=w134:refnum<vi>, error out=w133:errorcluster, "Value"=w136:u16)  [unwired: 1 in]
      n71 = Spreadsheet String To Array(format string="%s", spreadsheet string=w49, array type (2D Dbl)=string[] []) -> (array=w39:string[])  [unwired: 1 in]
      n72 = Build Array (concatenate)("--- Select all ---", w39) -> (w46:string[])
      n73 = property class="LstBox (strict)"(reference=w48, "Item Names"=w46) -> (reference out=w40:refnum<vi>, error out=w41:errorcluster, "Item Names"=w47:string[], "Value"=w32:i32[])  [unwired: 1 in]
      n74 = Equal?(x=w47, y=w46) -> (x = y?=w43:bool)
      n75 = Search 1D Array(1D array=w32, element=0) -> (index of element=w45:i32)  [unwired: 1 in]
      n76 = Greater Or Equal To 0?(x=w45) -> (x >= 0?=w44:bool)
      n77 = Array Size(array=w46) -> (size(s)=w62:i32)
      n78 = Compound Arithmetic op=OR(invert w43, w44) -> (w42:bool)
      n79 = case shown="True" w42 {
        tunnel: w40 -> [w212 w218]
        tunnel: w62 -> [_ w217]
        tunnel: [w212 w216] -> w61
        tunnel: w41 -> [w211 w215]
        tunnel: [w211 w214] -> w58
        frame False {
        }
        frame True {
          n80 = for {
            N: w217 -> [_]
            tunnel: [w219] -> w213 mode=indexing
            i -> [w220]
            n81 = Increment(x=w220) -> (x+1=w219:i32)
          }
          n82 = property class="LstBox (strict)"(reference=w218, error in=w215, "Value"=w213) -> (reference out=w216:refnum<vi>, error out=w214:errorcluster)
        }
      }
      n83 = property class="LstBox (strict)"(reference=w61, error in=w58) -> (error out=w57:errorcluster, "Value"=w60:i32[], "Item Names"=w59:string[])  [unwired: 1 out]
      n84 = call <vilib>:"Clear Errors.vi"("error in (no error)"=w57) -> ()  [unwired: 5 in, 2 out]
      n85 = for {
        tunnel: w60 -> [w209] mode=indexing
        tunnel: w59 -> [w210]
        tunnel: [w208] -> w37 mode=indexing
        n86 = Index Array(array=w210, index=w209) -> (element=w208:string)
      }
      n87 = Array Size(array=w138) -> (size(s)=w137:i32)
      n88 = Array To Spreadsheet String(delimiter (Tab)=", ", array=w37, 3:"'%s'" ("format string")) -> (spreadsheet string=w34:string)
      n89 = Format Into String(format string="Current: %s" ("delimiter (Tab)"), w66) -> (resulting string=w121:string)  [unwired: 2 in, 1 out]
      n90 = Greater Or Equal?(x=w136, y=w137) -> (x >= y?=w135:bool)
      n91 = call <vilib>:"Trim Whitespace.vi"("string"=w34) -> ("trimmed string"=w33:string)  [unwired: 1 in]
      n92 = case shown="True" w135 {
        tunnel: w134 -> [w254 w260]
        tunnel: w133 -> [w255 w259]
        tunnel: [w255 w257] -> w131
        tunnel: [w254 w256] -> w132
        frame False {
        }
        frame True {
          # "update chn selection\nif out of valid range"
          n93 = property class="Ring (strict)"(reference=w260, error in=w259, "Val(Sgnl)"=u16 0 ("Value")) -> (reference out=w256:refnum<vi>, error out=w257:errorcluster)
        }
      }
      n94 = Replace Array Subset(array=w69, new element=w121, index=0) -> (w114:string[])
      n95 = property class="Ring (strict)"(reference=w113, "Strings []"=w114) -> (reference out=w118:refnum<vi>, error out=w119:errorcluster, "Value"=w116:u16)  [unwired: 1 in]
      n96 = Compound Arithmetic op=AND(invert w55, w179) -> (w181:bool)
      n97 = Array Size(array=w114) -> (size(s)=w115:i32)
      n98 = Greater Or Equal?(x=w116, y=w115) -> (x >= y?=w117:bool)
      n99 = property class="DigNum (strict)"(reference=w173) -> (error out=w169:errorcluster, "Value"=w165:i32)  [unwired: 1 in, 1 out]
      n100 = case shown="True" w117 {
        tunnel: w118 -> [w247 w253]
        tunnel: w119 -> [w248 w252]
        tunnel: [w248 w250] -> _
        tunnel: [w247 w249] -> w112
        frame False {
        }
        frame True {
          # "update alg selection\nif out of valid range"
          n101 = property class="Ring (strict)"(reference=w253, error in=w252, "Val(Sgnl)"=u16 0 ("Value")) -> (reference out=w249:refnum<vi>, error out=w250:errorcluster)
        }
      }
      n102 = property class="Enum (strict)"(reference=w174) -> (error out=w170:errorcluster, "Value"=w166:T75)  [unwired: 1 in, 1 out]
      n103 = property class="Enum (strict)"(reference=w172) -> (error out=w168:errorcluster, "Value"=w164:T76)  [unwired: 1 in, 1 out]
      n104 = property class="Enum (strict)"(reference=w171) -> (error out=w167:errorcluster, "Value"=w163:T77)  [unwired: 1 in, 1 out]
      n105 = property class="Enum (strict)"(reference=w152) -> (error out=w153:errorcluster, "Value"=w151:T78)  [unwired: 1 in, 1 out]
      n106 = property class="Ring (strict)"(reference=w132, error in=w131) -> (error out=w148:errorcluster, "Value"=w147:u16)  [unwired: 1 out]
      n107 = property class="Ring (strict)"(reference=w177, error in=w178) -> (error out=w176:errorcluster, "Value"=w175:u16)  [unwired: 1 out]
      n108 = call <vilib>:"Clear Errors.vi"("error in (no error)"=w148) -> ()  [unwired: 5 in, 2 out]
      n109 = call <vilib>:"Clear Errors.vi"("error in (no error)"=w170) -> ()  [unwired: 5 in, 2 out]
      n110 = call <vilib>:"Clear Errors.vi"("error in (no error)"=w169) -> ()  [unwired: 5 in, 2 out]
      n111 = call <vilib>:"Clear Errors.vi"("error in (no error)"=w168) -> ()  [unwired: 5 in, 2 out]
      n112 = call <vilib>:"Clear Errors.vi"("error in (no error)"=w167) -> ()  [unwired: 5 in, 2 out]
      n113 = call <vilib>:"Clear Errors.vi"("error in (no error)"=w153) -> ()  [unwired: 5 in, 2 out]
      n114 = call <vilib>:"Clear Errors.vi"("error in (no error)"=w176) -> ()  [unwired: 5 in, 2 out]
      n115 = property class="Ring (strict)"(reference=w112) -> (error out=w110:errorcluster, "Value"=w111:u16)  [unwired: 1 in, 1 out]
      n116 = Unbundle By Name(w102) -> ("show graph"=w154:bool)
      n117 = call <vilib>:"Clear Errors.vi"("error in (no error)"=w110) -> ()  [unwired: 5 in, 2 out]
      n118 = Index Array(array=w69, index=w111) -> (element=w109:string)
      n119 = case shown="True" w181 {
        tunnel: w175 -> [_ w280]
        tunnel: w55 -> [w267 w286]
        tunnel: w166 -> [_ w285]
        tunnel: w165 -> [_ w284]
        tunnel: w164 -> [_ w283]
        tunnel: w163 -> [_ w282]
        tunnel: w80 -> [_ w281]
        tunnel: w53 -> [w264 w279]
        tunnel: w162 -> [w265 w278]
        tunnel: [w263 w277] -> w161
        tunnel: [w264 w276] -> w160
        tunnel: w84 -> [w261 w275]
        tunnel: [w261 w274] -> w64
        tunnel: w154 -> [_ w273]
        tunnel: w102 -> [_ w272]
        tunnel: w151 -> [_ w271]
        tunnel: w147 -> [_ w270]
        tunnel: w109 -> [_ w269]
        tunnel: w33 -> [_ w268]
        frame False {
          # "no result exist"
          n120 = call "Meas Proc QWTB String to Table Writter.vi"("param table ref"=w265, "error in"=w267, "force data update? (False)"=TRUE, "content csv string"="\nno results" ("control string")) -> ("error out"=w263:errorcluster)  [unwired: 6 in, 1 out]
        }
        frame True {
          # "some results exist, update"
          n121 = case shown="False" w273 {
            tunnel: w286 -> [w335 w357]
            tunnel: w285 -> [w333 _]
            tunnel: w284 -> [w332 _]
            tunnel: w283 -> [w331 _]
            tunnel: w282 -> [w330 _]
            tunnel: w281 -> [w329 w351]
            tunnel: w280 -> [w328 w356]
            tunnel: w279 -> [w327 w355]
            tunnel: w278 -> [w323 _]
            tunnel: [w318 w352] -> w277
            tunnel: [w317 w353] -> w276
            tunnel: w275 -> [w307 w349]
            tunnel: [w305 w349] -> w274
            tunnel: w272 -> [_ w342]
            tunnel: w271 -> [w290 w340]
            tunnel: w270 -> [w289 w339]
            tunnel: w269 -> [w288 w338]
            tunnel: w268 -> [w287 _]
            frame False {
              n122 = To Long Integer(number=w328) -> (32bit integer=w315:i32)
              n123 = Decrement(x=w315) -> (x-1=w316:i32)
              n124 = Format Into String(format string="cfg = struct();\ncfg.max_dim = %d;\ncfg.max_array = %d;\ncfg.group_mode = %d;\ncfg.unc_mode = %d;\ncfg.phi_mode = %d;\ncfg.phi_ref_chn = %d;\n[csv, desc, var_names, chn_id] = qwtb_get_results('%s', %d, '%s', cfg, {%s});", error in=w335, w333, w332, w331, w330, w290, w289, w329, w316, w288, w287) -> (resulting string=w337:string, error out=w336:errorcluster)  [unwired: 1 in]
              n125 = call "golpi_mpc_command.vi"("error in"=w336, "command"=w337, "GOLPI ref in"=w327) -> ("error out"=w324:errorcluster, "read buffer"=w325:string, "GOLPI ref. out"=w311:T73)  [unwired: 6 in]
              n126 = call "Check Output For Octave Errors.vi"("error in"=w324, "read buffer"=w325) -> ("error out"=w312:errorcluster)  [unwired: 9 in]
              n127 = call-poly "Get Variable.vi"("error in"=w312, "variable name"="desc", "GOLPI ref. in"=w311) -> ("error out"=w303:errorcluster, "value"=w310:string, "GOLPI ref. out"=w302:T73)  [unwired: 6 in]
              n128 = Spreadsheet String To Array(format string="%s", spreadsheet string=w310, array type (2D Dbl)=string[] []) -> (array=w306:string[])  [unwired: 1 in]
              n129 = call-poly "Get Variable.vi"("error in"=w303, "variable name"="var_names", "GOLPI ref. in"=w302) -> ("error out"=w297:errorcluster, "value"=w299:string, "GOLPI ref. out"=w296:T73)  [unwired: 6 in]
              n130 = Spreadsheet String To Array(format string="%s", spreadsheet string=w299, array type (2D Dbl)=string[] []) -> (array=w298:string[])  [unwired: 1 in]
              n131 = call-poly "Get Variable.vi"("error in"=w297, "variable name"="chn_id", "GOLPI ref. in"=w296) -> ("error out"=w295:errorcluster, "value"=w292:dbl[], "GOLPI ref. out"=w294:T73)  [unwired: 6 in]
              n132 = To Long Integer(number=w292) -> (32bit integer=w291:i32[])
              n133 = call-poly "Get Variable.vi"("error in"=w295, "variable name"="csv", "GOLPI ref. in"=w294) -> ("error out"=w322:errorcluster, "value"=w320:string, "GOLPI ref. out"=w317:T73)  [unwired: 6 in]
              n134 = Bundle By Name(cluster=w307, "channel indexes"=w291, "var names"=w298, "descriptions"=w306) -> (w305:T69)
              n135 = Select(t="\nerror", s=w322, f=w320) -> (s? t:f=w321:string)
              n136 = call "Meas Proc QWTB String to Table Writter.vi"("param table ref"=w323, "error in"=w322, "force data update? (False)"=TRUE, "content csv string"=w321) -> ("error out"=w318:errorcluster)  [unwired: 6 in, 1 out]
            }
            frame True {
              n137 = To Long Integer(number=w356) -> (32bit integer=w354:i32)
              n138 = Decrement(x=w354) -> (x-1=w350:i32)
              n139 = Unbundle By Name(w349) -> ("channel indexes"=w341:i32[], "var names"=w343:string[], "qwtb results tbl"=w348:refnum<vi>)
              n140 = property class="Tbl (strict)"(reference=w348) -> ("Selection Size"=w347:T79, "Selection Start"=w346:T79)  [unwired: 1 in, 2 out]
              n141 = Unbundle By Name(w347) -> ("Row"=w345:i32)
              n142 = Unbundle By Name(w346) -> ("Row"=w344:i32)
              n143 = case shown="Default" w345 {
                tunnel: w357 -> [w359 w390]
                tunnel: w355 -> [w358 w380]
                tunnel: [w358 w386] -> w353
                tunnel: [w359 w385] -> w352
                tunnel: w351 -> [_ w384]
                tunnel: w350 -> [_ w383]
                tunnel: w344 -> [_ w367]
                tunnel: w343 -> [_ w382]
                tunnel: w342 -> [_ w379]
                tunnel: w341 -> [_ w368]
                tunnel: w340 -> [_ w362]
                tunnel: w339 -> [_ w361]
                tunnel: w338 -> [_ w360]
                frame 0 {
                }
                frame Default {
                  n144 = Unbundle By Name(w379) -> ("plot setup.show all chn"=w366:bool, "plot setup.Show legend"=w373:T1, "plot setup.X-axis style"=w378:T72, "plot setup.Y-axis style"=w377:T72, "plot setup.Box on"=w376:bool, "plot setup.Grid on"=w375:bool)
                  n145 = Index Array(array=w368, index=w367) -> (element=w365:i32)
                  n146 = Index Array(array=w382, index=w367) -> (element=w381:string)
                  n147 = property on="Show legend" class="Enum (strict)"() -> ("Strings []"=w374:string[])  [unwired: 2 in, 2 out]
                  n148 = Select(t=0, s=w366, f=w365) -> (s? t:f=w363:i32)
                  n149 = Index Array(array=w374, index=w373) -> (element=w371:string)
                  n150 = Equal To 0?(x=w373) -> (x = 0?=w372:bool)
                  n151 = Select(t="", s=w372, f=w371) -> (s? t:f=w369:string)
                  n152 = Format Into String(format string="gcfg = struct();\ngcfg.xlog = %d;\ngcfg.ylog = %d;\ngcfg.box = %d;\ngcfg.grid = %d;\ngcfg.legend = '%s';\ncfg = struct();\ncfg.phi_mode = %d;\ncfg.phi_ref_chn = %d;\nqwtb_plot_result('%s', %d, '%s', %d, cfg, '%s', gcfg);", error in=w390, w378, w377, w376, w375, w369, w362, w361, w384, w383, w360, w363, w381) -> (resulting string=w392:string, error out=w391:errorcluster)  [unwired: 1 in]
                  n153 = call "golpi_mpc_command.vi"("error in"=w391, "command"=w392, "GOLPI ref in"=w380) -> ("error out"=w387:errorcluster, "read buffer"=w388:string, "GOLPI ref. out"=w386:T73)  [unwired: 6 in]
                  n154 = call "Check Output For Octave Errors.vi"("error in"=w387, "read buffer"=w388) -> ("error out"=w385:errorcluster)  [unwired: 9 in]
                }
              }
            }
          }
        }
      }
      n155 = call "golpi_mpc_release.vi"("error in"=w161, "golpi ref or golpi session in"=w160, "golpi session ref"=w159) -> ("error out"=w72:errorcluster)  [unwired: 7 in, 1 out]
      n156 = Select(t="<tc=red><b>Error!" ("string (empty)"), s=w72, f="<tc=green><b>Ready" ("string (empty)")) -> (s? t:f=w71:string)
    }
  }
  n157 = Unbundle By Name(w2) -> ("qwtb results tbl"=w1:refnum<vi>)
  n158 = call-poly "SGUI Assign String With Tags.vi"("error in"=w6, "label(s) (empty)"="qwtb res info", "string (empty)"=w5) -> ("error out"=w4:errorcluster)  [unwired: 7 in, 1 out]
  n159 = To Variant(anything=w2) -> (Variant=→"QWTB result session out":variant)
  n160 = case shown="Error" w4 {
    selector: w4 -> [w400 w404]
    tunnel: [w400 w403] -> w3
    tunnel: w1 -> [_ w402]
    frame No Error {
    }
    frame Error {
      # "clear table when error occures"
      n161 = call "Meas Proc QWTB String to Table Writter.vi"("param table ref"=w402, "force data update? (False)"=TRUE) -> ("error out"=w405:errorcluster)  [unwired: 8 in, 1 out]
      n162 = Merge Errors(w404, w405) -> (w403:errorcluster)
    }
  }
  "error out" <- w3
